vi "Main.vi"() -> ()   [LabVIEW 2012]
panel:
  in  "Drive Error":errorcluster
  in  "Torsion Error":errorcluster
  in  "IMU Error":errorcluster
  in  "Drive VISA":refnum<visa-resource-name>
  in  "Torsion VISA":refnum<visa-resource-name>
  in  "IMU VISA":refnum<visa-resource-name>
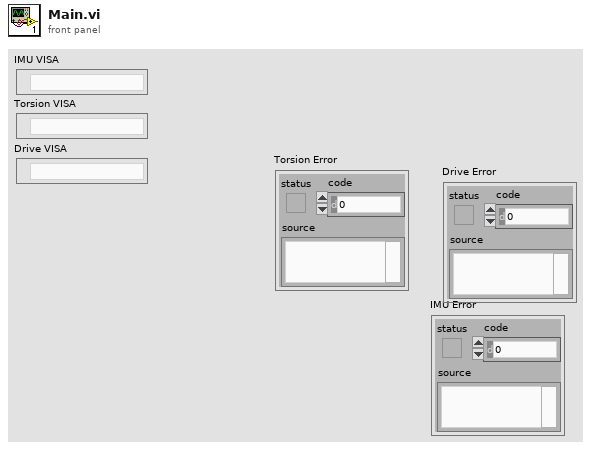
[diagram p1: front panel]
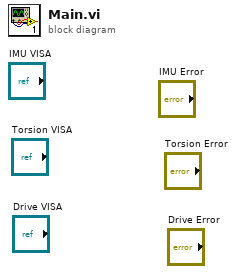
[diagram p0: block diagram]
diagram:
